vi "SP Set Display Formats.vi"(8 "error in (no error)":errorcluster, 10 "Format":T1 caption="Display Format" items=["Log Mag", "Phase", "Expanded Phase", "Delay", "Smith", "Polar", "Lin Mag", "SWR", "Loss", "Real", "Imaginary"], 11 "CH Controls":T2={"Trace On"=TRUE, "Measure"=0, "Format"=0, "Autoscale"=TRUE, "Reference"=0.0, "\nRefUnit"="dB/Div", "Position"=5.0, "Scale"=10.0, "ScaleUnit"="dB/Div", "LimitOn"=TRUE, "LimitFill"=FALSE, "Display Data"=0, "Show Markers"=TRUE, "SXX"=""} {"Reference" format="%#.2g"; "Display Data" items=["Data", "Memory", "Data/Memory"]; "Format" items=["Log Mag", "Phase", "Expanded Phase", "Delay", "Smith", "Polar", "Lin Mag", "SWR", "Loss", "Real", "Imaginary"]; "Scale" min=0.001 step=1.0 format="%#.2g"; "Position" min=0.0 max=10.0}) -> (0 "error out":errorcluster, 3 "new CH Controls":T2={"Trace On"=TRUE, "Measure"=0, "Format"=0, "Autoscale"=TRUE, "Reference"=0.0, "\nRefUnit"="dB/Div", "Position"=5.0, "Scale"=10.0, "ScaleUnit"="dB/Div", "LimitOn"=TRUE, "LimitFill"=FALSE, "Display Data"=0, "Show Markers"=TRUE, "SXX"=""} {"Reference" format="%#.2g"; "Display Data" items=["Data", "Memory", "Data/Memory"]; "Format" items=["Log Mag", "Phase", "Expanded Phase", "Delay", "Smith", "Polar", "Lin Mag", "SWR", "Loss", "Real", "Imaginary"]; "Scale" min=0.001 step=1.0 format="%#.2g"; "Position" min=0.0 max=10.0})   [LabVIEW 2011]
uses:
  TypeDefs/SP Display Trace Controls.ctl
  TypeDefs/SP Display Format.ctl
  TypeDefs/SP Display Data.ctl
panel:
  # "Div"
  # "Div"
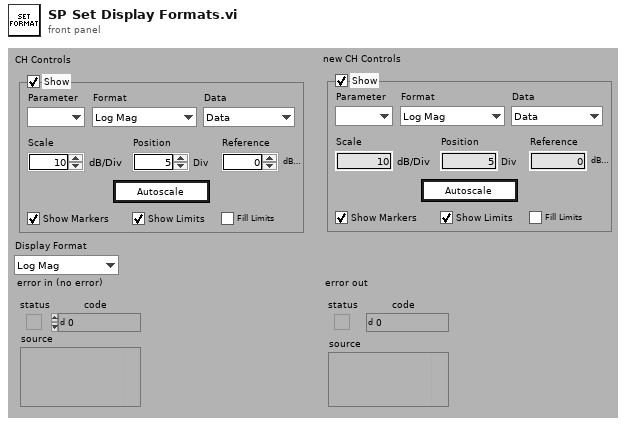
[diagram p1: front panel]
types:
  T1 = typedef "SP Display Format.ctl" = i32
  T2 = typedef "SP Display Trace Controls.ctl" = cluster{"Trace On":bool, "Measure":i32, "Format":T1, "Autoscale":bool, "Reference":dbl, "\nRefUnit":string, "Position":dbl, "Scale":dbl, "ScaleUnit":string, "LimitOn":bool, "LimitFill":bool, "Display Data":T3, "Show Markers":bool, "SXX":string}
  T3 = typedef "SP Display Data.ctl" = u16
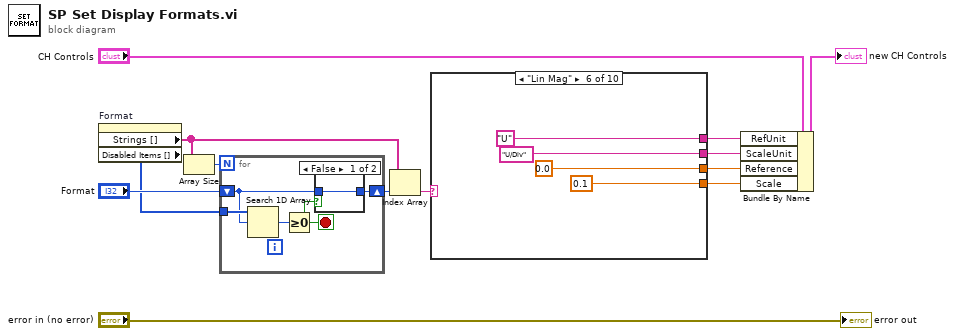
[diagram p0: block diagram]
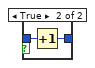
[diagram p2: hidden frame]
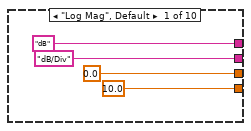
[diagram p3: hidden frame]
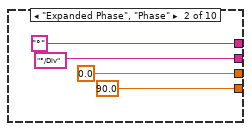
[diagram p4: hidden frame]
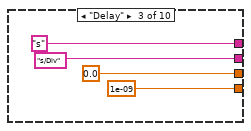
[diagram p5: hidden frame]
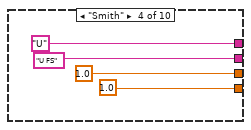
[diagram p6: hidden frame]
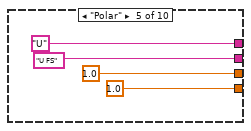
[diagram p7: hidden frame]
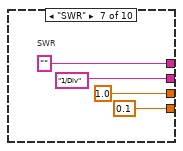
[diagram p8: hidden frame]
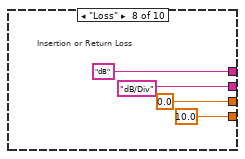
[diagram p9: hidden frame]
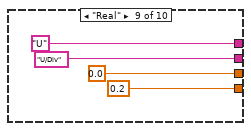
[diagram p10: hidden frame]
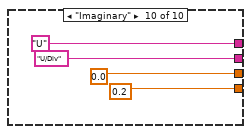
[diagram p11: hidden frame]
diagram:
  n1 = property on="Format" class="Ring (strict)"() -> ("Strings []"=w3:string[], "Disabled Items []"=w4:i32[])  [unwired: 2 in, 2 out]
  n2 = Array Size(array=w3) -> (size(s)=w1:i32)
  n3 = for {
    N: w1 -> [_]
    tunnel: w4 -> [w18]
    shift-right: [w15] -> w2
    shift-left: "Format" -> [w16]
    stop <- w14 stop-if-true
    n4 = Search 1D Array(1D array=w18, element=w16) -> (index of element=w17:i32)  [unwired: 1 out]
    n5 = Greater Or Equal To 0?(x=w17) -> (x >= 0?=w14:bool)
    n6 = case shown="False" w14 {
      tunnel: w16 -> [w19 w21]
      tunnel: [w19 w20] -> w15
      frame False {
      }
      frame True {
        n7 = Increment(x=w21) -> (x+1=w20:T1)
      }
    }
  }
  n8 = Index Array(array=w3, index=w2) -> (element=w6:string)
  n9 = case shown="\"Lin Mag\"" w6 {
    tunnel: ["dB" "°" "s" "U" "U" "U" "" "dB" "U" "U"] -> w13
    tunnel: ["dB/Div" "°/Div" "s/Div" "U FS" "U FS" "U/Div" "1/Div" "dB/Div" "U/Div" "U/Div"] -> w12
    tunnel: [0.0 ("Reference") 0.0 ("Reference") 0.0 ("Reference") 1.0 ("Reference") 1.0 ("Reference") 0.0 ("Reference") 1.0 ("Reference") 0.0 ("Reference") 0.0 ("Reference") 0.0 ("Reference")] -> w9
    tunnel: [10.0 ("Reference") 90.0 ("Reference") 1e-09 ("Reference") 1.0 ("Reference") 1.0 ("Reference") 0.1 ("Reference") 0.1 ("Reference") 10.0 ("Reference") 0.2 ("Reference") 0.2 ("Reference")] -> w8
    frame "Log Mag", Default {
    }
    frame "Expanded Phase", "Phase" {
    }
    frame "Delay" {
    }
    frame "Smith" {
    }
    frame "Polar" {
    }
    frame "Lin Mag" {
    }
    frame "SWR" {
      # "SWR"
    }
    frame "Loss" {
      # "Insertion or Return Loss"
    }
    frame "Real" {
    }
    frame "Imaginary" {
    }
  }
  n10 = Bundle By Name(cluster="CH Controls", "RefUnit"=w13, "ScaleUnit"=w12, "Reference"=w9, "Scale"=w8) -> (→"new CH Controls":T2)
  "error out" <- "error in (no error)"
